vi "RequiredForLvNative-InstrumentAction.vi"(7 "action":string, 8 "error in (no error)":errorcluster, 10 "Parameter":variant, 11 "CAN-NI in":refnum<class "CAN-NI.lvclass">) -> (0 "error out":errorcluster, 2 "Result":variant, 3 "CAN-NI out":refnum<class "CAN-NI.lvclass">)   [LabVIEW 2019, in "CAN-NI.lvlib" / "CAN-NI.lvclass"]
uses:
  CAN-NI.lvclass
  CAN-Interface/TypeDef/Def-PreConfig-BaudRate.ctl
  CAN-Interface/TypeDef/Def-BaudRate.ctl
  CAN-Interface/TypeDef/Def-PreConfig-Termination.ctl
  CAN-Interface/TypeDef/Def-Termination.ctl
  CAN-Interface/TypeDef/Def-OpenDevice.ctl
  CAN-Interface/TypeDef/Def-TransmitData.ctl
  CAN-Interface/TypeDef/Def-CANData.ctl
  CAN-Interface/TypeDef/Def-ReceiveData.ctl
  CAN-Interface/Class-Interface.lvclass
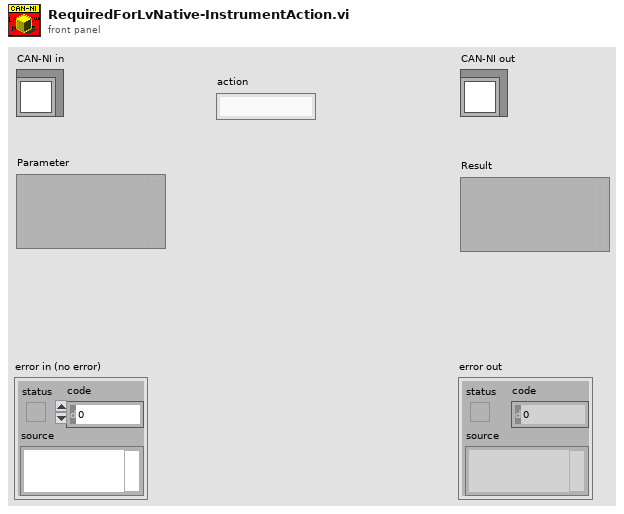
[diagram p1: front panel]
types:
  T1 = typedef "CAN-Interface.lvlib/Class-Interface.lvclass/Def-PreConfig-BaudRate.ctl" = cluster{"Channel Num":u32, "BaudRate":T2}
  T2 = typedef "CAN-Interface.lvlib/Class-Interface.lvclass/Def-BaudRate.ctl" = u32
  T3 = typedef "CAN-Interface.lvlib/Class-Interface.lvclass/Def-PreConfig-Termination.ctl" = cluster{"Channel Num":u32, "Termination":T4}
  T4 = typedef "CAN-Interface.lvlib/Class-Interface.lvclass/Def-Termination.ctl" = enum8{"on", "off"}
  T5 = typedef "CAN-Interface.lvlib/Class-Interface.lvclass/Def-OpenDevice.ctl" = cluster{"DeviceType":string, "DeviceIndex":u32}
  T6 = typedef "CAN-Interface.lvlib/Class-Interface.lvclass/Def-TransmitData.ctl" = cluster{"Channel Num":u32, "FrameData":T7}
  T7 = typedef "CAN-Interface.lvlib/Class-Interface.lvclass/Def-CANData.ctl" = cluster{"Identifier":u32, "PayLoad":u8[]}
  T8 = typedef "CAN-Interface.lvlib/Class-Interface.lvclass/Def-ReceiveData.ctl" = cluster{"Channel Num":u32, "timeout(ms)":i32}
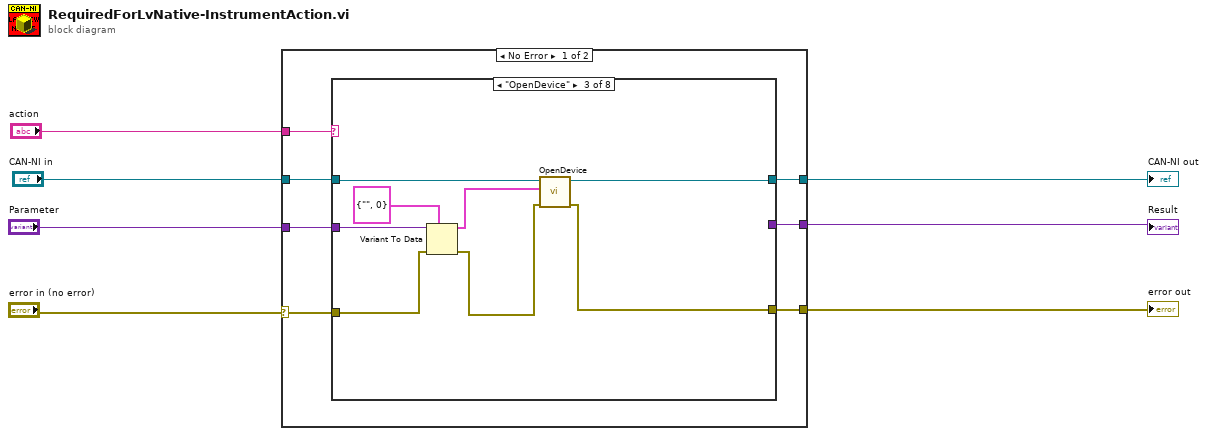
[diagram p0: block diagram]
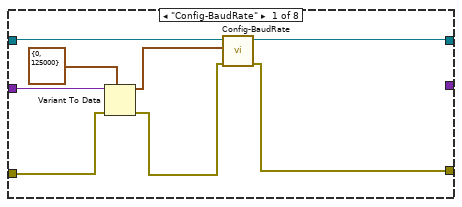
[diagram p2: hidden frame]
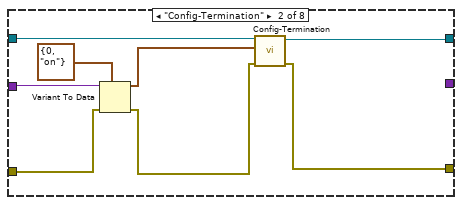
[diagram p3: hidden frame]
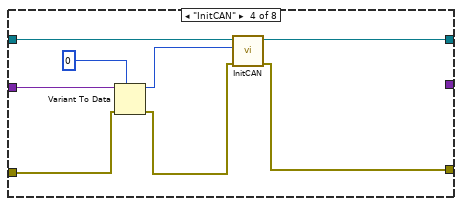
[diagram p4: hidden frame]
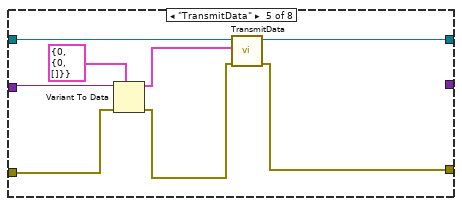
[diagram p5: hidden frame]
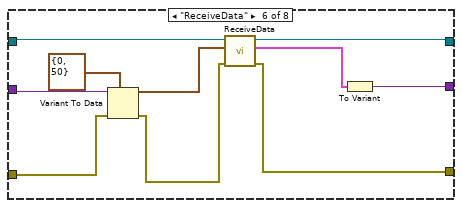
[diagram p6: hidden frame]
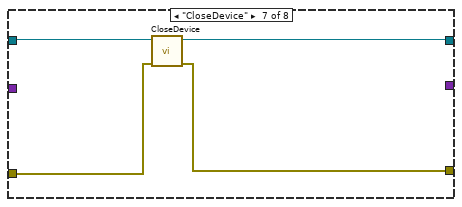
[diagram p7: hidden frame]
diagram:
  n1 = case shown="No Error" "error in (no error)" {
    selector: "error in (no error)" -> [w10 w72]
    tunnel: "action" -> [w14 _]
    tunnel: "CAN-NI in" -> [w13 w71]
    tunnel: [w12 w71] -> w5
    tunnel: "Parameter" -> [w11 _]
    tunnel: [w9 w72] -> w2
    tunnel: [w8 _] -> w1
    frame No Error {
      n2 = case shown="\"OpenDevice\"" w14 {
        tunnel: w13 -> [w19 w27 w35 w43 w51 w61 w68 w70]
        tunnel: [w16 w26 w32 w42 w47 w60 w66 w70] -> w12
        tunnel: w11 -> [w21 w30 w38 w46 w54 w64 _ _]
        tunnel: w10 -> [w22 w29 w37 w45 w53 w63 w67 w69]
        tunnel: [w17 w23 w31 w40 w48 w58 w65 w69] -> w9
        tunnel: [_ _ _ _ _ w56 _ _] -> w8
        frame "Config-BaudRate" {
          n3 = Variant To Data(error in=w22, type=T1 {"Channel Num"=0, "BaudRate"=125000} ("Def-PreConfig-BaudRate"), Variant=w21) -> (data=w15:T1, error out=w18:errorcluster)
          n4 = call-dynamic "Config-BaudRate.vi"("error in (no error)"=w18, "Def-PreConfig-BaudRate"=w15, "CAN-NI in"=w19) -> ("error out"=w17:errorcluster, "CAN-NI out"=w16:refnum<class "CAN-NI.lvclass">)  [unwired: 7 in]
        }
        frame "Config-Termination" {
          n5 = Variant To Data(error in=w29, type=T3 {"Channel Num"=0, "Termination"=enum."on"} ("Def-PreConfig-Termination"), Variant=w30) -> (data=w24:T3, error out=w25:errorcluster)
          n6 = call-dynamic "Config-Termination.vi"("error in (no error)"=w25, "Def-PreConfig-Termination"=w24, "CAN-NI in"=w27) -> ("error out"=w23:errorcluster, "CAN-NI out"=w26:refnum<class "CAN-NI.lvclass">)  [unwired: 7 in]
        }
        frame "OpenDevice" {
          n7 = Variant To Data(error in=w37, type=T5 {"DeviceType"="", "DeviceIndex"=0} ("Def-OpenDevice"), Variant=w38) -> (data=w34:T5, error out=w33:errorcluster)
          n8 = call-dynamic "OpenDevice.vi"("error in (no error)"=w33, "Def-OpenDevice"=w34, "CAN-NI in"=w35) -> ("error out"=w31:errorcluster, "CAN-NI out"=w32:refnum<class "CAN-NI.lvclass">)  [unwired: 7 in]
        }
        frame "InitCAN" {
          n9 = Variant To Data(error in=w45, type=u32 0, Variant=w46) -> (data=w39:u32, error out=w41:errorcluster)
          n10 = call-dynamic "InitCAN.vi"("error in (no error)"=w41, "Channel Num"=w39, "CAN-NI in"=w43) -> ("error out"=w40:errorcluster, "CAN-NI out"=w42:refnum<class "CAN-NI.lvclass">)  [unwired: 7 in]
        }
        frame "TransmitData" {
          n11 = Variant To Data(error in=w53, type=T6 {"Channel Num"=0, "FrameData"={"Identifier"=0, "PayLoad"=[]}} ("Def-TransmitData"), Variant=w54) -> (data=w50:T6, error out=w49:errorcluster)
          n12 = call-dynamic "TransmitData.vi"("error in (no error)"=w49, "Def-TransmitData"=w50, "CAN-NI in"=w51) -> ("error out"=w48:errorcluster, "CAN-NI out"=w47:refnum<class "CAN-NI.lvclass">)  [unwired: 7 in]
        }
        frame "ReceiveData" {
          n13 = Variant To Data(error in=w63, type=T8 {"Channel Num"=0, "timeout(ms)"=50} ("Def-ReceiveData"), Variant=w64) -> (data=w57:T8, error out=w59:errorcluster)
          n14 = call-dynamic "ReceiveData.vi"("error in (no error)"=w59, "Def-ReceiveData"=w57, "CAN-NI in"=w61) -> ("error out"=w58:errorcluster, "FrameData"=w55:T7, "CAN-NI out"=w60:refnum<class "CAN-NI.lvclass">)  [unwired: 6 in]
          n15 = To Variant(anything=w55) -> (Variant=w56:variant)
        }
        frame "CloseDevice" {
          n16 = call-dynamic "CloseDevice.vi"("error in (no error)"=w67, "CAN-NI in"=w68) -> ("error out"=w65:errorcluster, "CAN-NI out"=w66:refnum<class "CAN-NI.lvclass">)  [unwired: 8 in]
        }
        frame Default {
        }
      }
    }
    frame Error {
    }
  }
  "error out" <- w2
  "CAN-NI out" <- w5
  "Result" <- w1
